vi "Lorentz fit normal and dispersive.vi"(6 "cursor diff":dbl, 9 "cursor avg":dbl, 10 "Y subset":dbl[](array[numeric]), 11 "X subset":dbl[](array[numeric])) -> (0 "error out":errorcluster, 1 "Initial params":dbl[](array[numeric]), 2 "best fit parameters":dbl[](array[numeric]), 3 "best nonlinear fit":dbl[](array[numeric]))   [LabVIEW 2015]
panel:
  # "Fitting to a more complicated Lorentzian-like function\n(called \"lfun3c\" in my Matlab functions):\nF = p(1)./((x-p(2)).^2+(p(3)^2)) + p(4)"
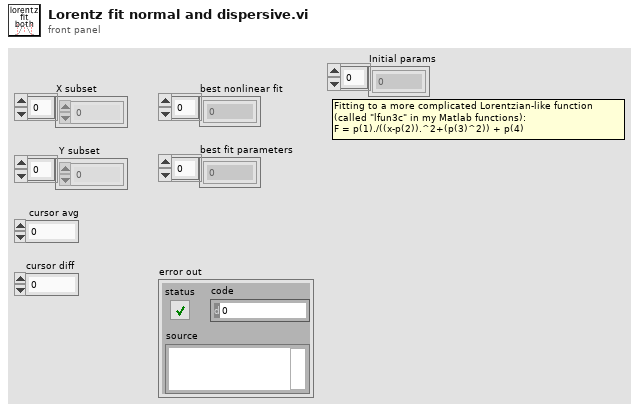
[diagram p1: front panel]
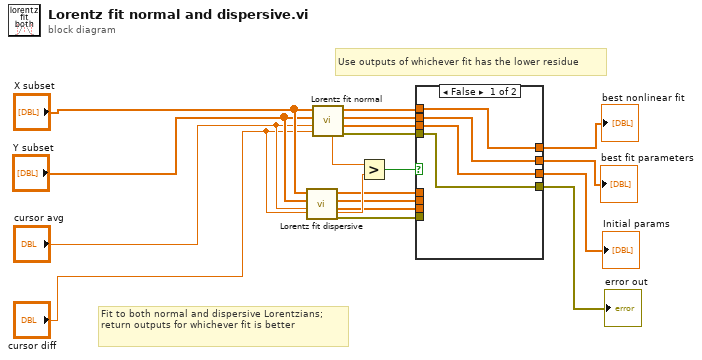
[diagram p0: block diagram]
diagram:
  # "Use outputs of whichever fit has the lower residue"
  # "Fit to both normal and dispersive Lorentzians;\nreturn outputs for whichever fit is better"
  n1 = call "Lorentz fit dispersive.vi"("cursor diff"="cursor diff", "cursor avg"="cursor avg", "Y subset"="Y subset", "X subset"="X subset") -> ("error out"=w9:errorcluster, "Initial params"=w10:dbl[], "best fit parameters"=w11:dbl[], "best nonlinear fit"=w12:dbl[], "residue"=w14:dbl)  [unwired: 3 in]
  n2 = call "Lorentz fit normal.vi"("cursor diff"="cursor diff", "cursor avg"="cursor avg", "Y subset"="Y subset", "X subset"="X subset") -> ("error out"=w5:errorcluster, "Initial params"=w6:dbl[], "best fit parameters"=w7:dbl[], "best nonlinear fit"=w8:dbl[], "residue"=w15:dbl)  [unwired: 3 in]
  n3 = Greater?(x=w15, y=w14) -> (0:w13:bool)
  n4 = case shown="False" w13 {
    tunnel: w12 -> [_ w27]
    tunnel: w11 -> [_ w26]
    tunnel: w10 -> [_ w25]
    tunnel: w9 -> [_ w24]
    tunnel: w8 -> [w23 _]
    tunnel: w7 -> [w22 _]
    tunnel: w6 -> [w21 _]
    tunnel: w5 -> [w20 _]
    tunnel: [w23 w27] -> w4
    tunnel: [w22 w26] -> w3
    tunnel: [w21 w25] -> w2
    tunnel: [w20 w24] -> w1
    frame False {
    }
    frame True {
    }
  }
  "error out" <- w1
  "best fit parameters" <- w3
  "best nonlinear fit" <- w4
  "Initial params" <- w2
